vi "update_weight_j.vi"(0 "w_jk_1":dbl, 1 "O_k":dbl, 2 "O_k 2":dbl, 3 "O_k 3":dbl, 4 "etta":dbl, 5 "w_jk_2":dbl, 6 "O_(L-1)":dbl, 7 "w_jk_3":dbl, 9 "O_j":dbl, 12 "t_k":dbl, 13 "t_k 2":dbl, 14 "t_k 3":dbl) -> (15 "w":dbl)   [LabVIEW 2014]
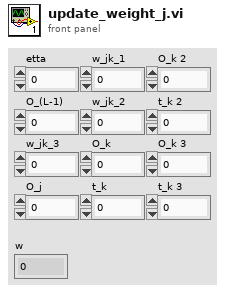
[diagram p1: front panel]
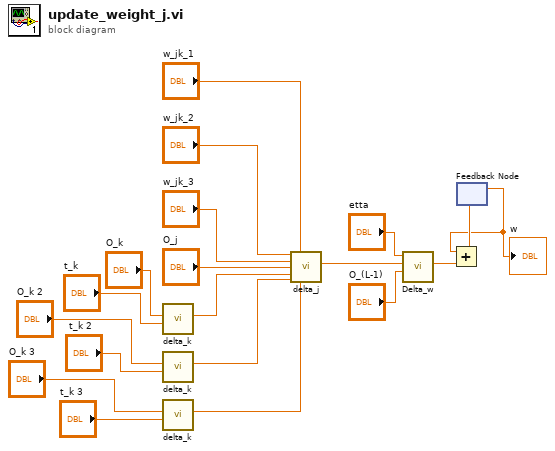
[diagram p0: block diagram]
diagram:
  n1 = call "delta_k.vi"("t_k"="t_k", "O_k"="O_k") -> ("delta_k"=w13:dbl)  [unwired: 9 in]
  n2 = call "delta_k.vi"("t_k"="t_k 2", "O_k"="O_k 2") -> ("delta_k"=w12:dbl)  [unwired: 9 in]
  n3 = call "delta_k.vi"("t_k"="t_k 3", "O_k"="O_k 3") -> ("delta_k"=w11:dbl)  [unwired: 9 in]
  n4 = call "delta_j.vi"("w_jk_2"="w_jk_2", "w_jk_1"="w_jk_1", "w_jk_3"="w_jk_3", "O_j"="O_j", "delta_k_1"=w13, "delta_k_2"=w12, "delta_k_3"=w11) -> ("delta_j"=w16:dbl)  [unwired: 8 in]
  n5 = call "Delta_w.vi"("O_(L-1)"="O_(L-1)", "Delta_L"=w16, "etta"="etta") -> ("Delta_w"=w17:dbl)  [unwired: 8 in]
  n6 = feedback #1() -> (w18:dbl)  [unwired: 1 in]
  "w" <- w18
  n7 = Add(x=w18, y=w17) -> (x+y=w19:dbl)
  n8 = feedback-in #1(w19) -> ()
